vi "camera mode cube.vi"   [LabVIEW 2018]
uses:
  ARM angles.vi
types:
  T1 = enum16{"shoulder", "elbow", "wrist", "base", "gripper"}
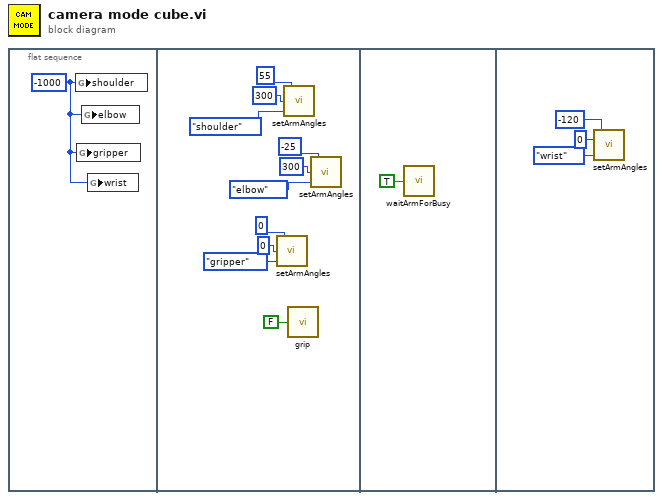
[diagram p0: block diagram]
diagram:
  n1 = flat-sequence {
    frame #0 {
      w1 = -1000 ("shoulder")
      n2 = global write "ARM angles.vi" "shoulder"(w1) -> ()
      n3 = global write "ARM angles.vi" "gripper"(w1) -> ()
      n4 = global write "ARM angles.vi" "elbow"(w1) -> ()
      n5 = global write "ARM angles.vi" "wrist"(w1) -> ()
    }
    frame #1 {
      n6 = call "setArmAngles.vi"("Enum"=T1."gripper", "speed"=0, "angle"=0) -> ()  [unwired: 1 in]
      n7 = call "setArmAngles.vi"("Enum"=T1."shoulder", "speed"=300, "angle"=55) -> ()  [unwired: 1 in]
      n8 = call "grip.vi"("grip"=FALSE) -> ()
      n9 = call "setArmAngles.vi"("Enum"=T1."elbow", "speed"=300, "angle"=-25) -> ()  [unwired: 1 in]
    }
    frame #2 {
      n10 = call "waitArmForBusy.vi"("base"=TRUE) -> ()
    }
    frame #3 {
      n11 = call "setArmAngles.vi"("Enum"=T1."wrist", "speed"=0, "angle"=-120) -> ()  [unwired: 1 in]
    }
  }
